vi "GlobalBatteryVoltageID.vi"() -> ()   [LabVIEW 2015]
panel:
  out "Batt Voltage ID":dbl
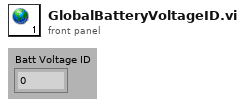
[diagram p1: front panel]
diagram:
